vi "TDMS Find Data File.vi"(8 "error in (no error)":errorcluster, 9 "Test Type":string, 10 "Serial Number":string, 11 "Model Number":string) -> (0 "error out":errorcluster, 2 "Found?":bool, 3 "TDMS Path":path)   [LabVIEW 2011]
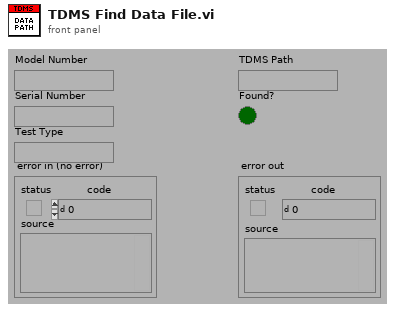
[diagram p1: front panel]
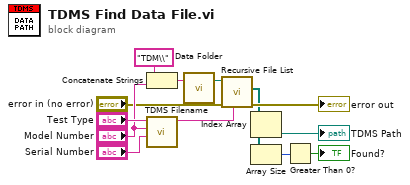
[diagram p0: block diagram]
diagram:
  n1 = Concatenate Strings("TDM\\" ("Relative Path (\"\" - Folder)"), "Model Number") -> (w10:string)
  n2 = call "TDMS Filename.vi"("Serial Number"="Serial Number", "Model Number"="Model Number", "Test Type"="Test Type") -> ("Filename"=w5:string)  [unwired: 8 in]
  n3 = call "Data Folder.vi"("Relative Path (\"\" - Folder)"=w10) -> ("Data Folder"=w6:path)  [unwired: 2 in]
  n4 = call <vilib>:"Recursive File List.vi"("pattern"=w5, "error in (no error)"="error in (no error)", "Folder Path"=w6) -> ("error out"=→"error out":errorcluster, "All Files in Dir"=w2:path[])  [unwired: 4 in, 3 out]
  n5 = Index Array(array=w2) -> (element=→"TDMS Path":path)  [unwired: 1 in]
  n6 = Array Size(array=w2) -> (size(s)=w3:i32)
  n7 = Greater Than 0?(x=w3) -> (x > 0?=→"Found?":bool)
